vi "Vertical X Axis.vi"() -> ()   [LabVIEW 2011]
panel:
  in  "stop":bool
  in  "Numeric 5":dbl caption="4.000000"
  in  "Numeric 4":dbl caption="3.000000"
  in  "Numeric 3":dbl caption="2.000000"
  in  "Numeric 2":dbl caption="1.000000"
  in  "Numeric":dbl caption="0.000000"
  out "Waveform Chart":dbl(graph)
  # "Hidden off-screen"
  # "Place the controls whose captions you are using for the x axis off the screen. Do not hide them, or the caption will be hidden as well. If you have existing controls, you can use their captions, since doing so will not interfere with the control value itself."
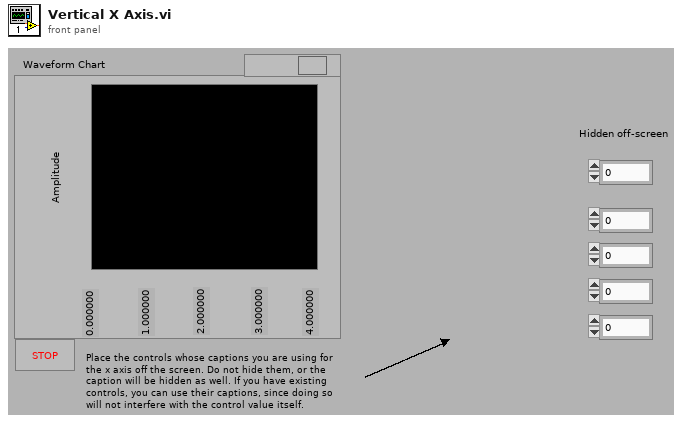
[diagram p1: front panel]
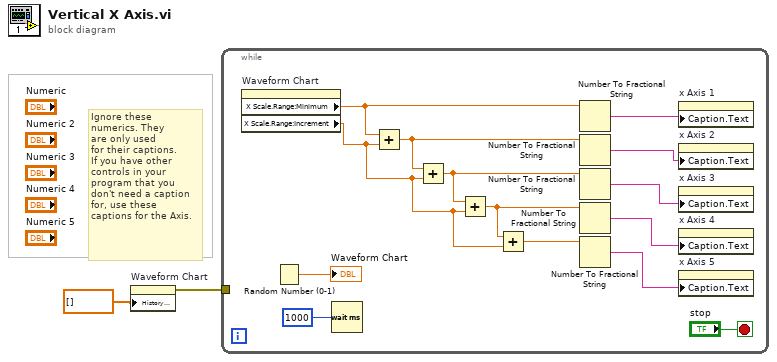
[diagram p0: block diagram]
diagram:
  # "Ignore these\nnumerics. They\nare only used \nfor their captions.\nIf you have other\ncontrols in your \nprogram that you\ndon't need a caption\nfor, use these \ncaptions for the Axis."
  n1 = property on="Waveform Chart" class="WFChart (strict)"("History Data"=dbl[] []) -> (error out=w1:errorcluster)  [unwired: 2 in, 1 out]
  n2 = while {
    tunnel: w1 -> [_]
    stop <- "stop" stop-if-true
    n3 = property on="Waveform Chart" class="WFChart (strict)"() -> ("X Scale.Range:Minimum"=w8:dbl, "X Scale.Range:Increment"=w7:dbl)  [unwired: 2 in, 2 out]
    n4 = Random Number (0-1)() -> (number: 0 to 1=→"Waveform Chart":dbl)
    n5 = Wait (ms)(milliseconds to wait=u32 1000) -> ()  [unwired: 1 out]
    n6 = Add(x=w8, y=w7) -> (x+y=w3:dbl)
    n7 = Add(x=w3, y=w7) -> (x+y=w4:dbl)
    n8 = Add(x=w4, y=w7) -> (x+y=w5:dbl)
    n9 = Add(x=w5, y=w7) -> (x+y=w6:dbl)
    n10 = Number To Fractional String(number=w8) -> (F-format string=w16:string)  [unwired: 3 in]
    n11 = Number To Fractional String(number=w3) -> (F-format string=w15:string)  [unwired: 3 in]
    n12 = Number To Fractional String(number=w4) -> (F-format string=w14:string)  [unwired: 3 in]
    n13 = Number To Fractional String(number=w5) -> (F-format string=w13:string)  [unwired: 3 in]
    n14 = Number To Fractional String(number=w6) -> (F-format string=w12:string)  [unwired: 3 in]
    n15 = property on="x Axis 1" class="DigNum (strict)"("Caption.Text"=w16) -> ()  [unwired: 2 in, 2 out]
    n16 = property on="x Axis 2" class="DigNum (strict)"("Caption.Text"=w15) -> ()  [unwired: 2 in, 2 out]
    n17 = property on="x Axis 3" class="DigNum (strict)"("Caption.Text"=w14) -> ()  [unwired: 2 in, 2 out]
    n18 = property on="x Axis 4" class="DigNum (strict)"("Caption.Text"=w13) -> ()  [unwired: 2 in, 2 out]
    n19 = property on="x Axis 5" class="DigNum (strict)"("Caption.Text"=w12) -> ()  [unwired: 2 in, 2 out]
  }
